vi "Event Demo.vi"() -> ()   [LabVIEW 2020]
uses:
  Flex/Flex.lvlib
  Flex/Element.ctl
  Flex/Event Data.ctl
panel:
  in  "Stop":bool
  in  "Slide":dbl(slide) scale=0.0..10.0
  out "Chart":dbl(graph)
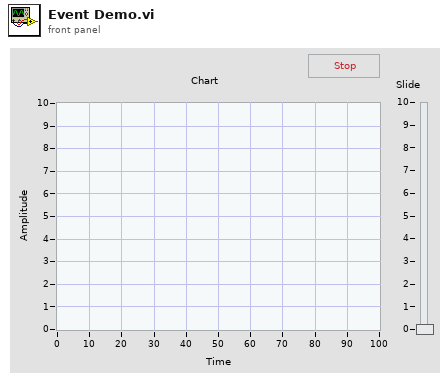
[diagram p1: front panel]
types:
  T1 = typedef "Flex.lvlib/))Channel.ctl" = refnum<queue>
  T2 = typedef "Flex.lvlib/Element.ctl" = dbl
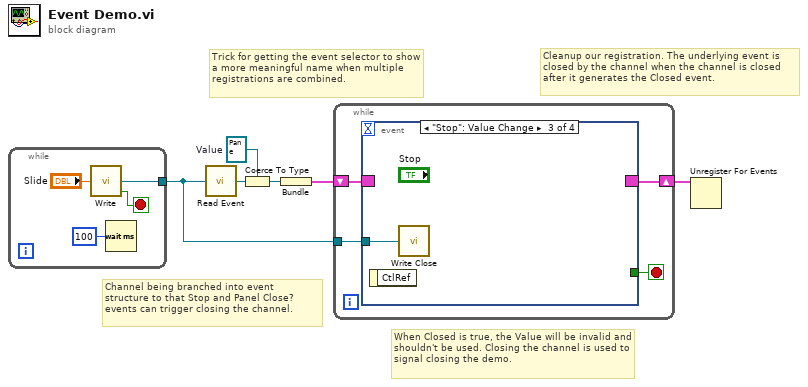
[diagram p0: block diagram]
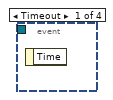
[diagram p2: hidden frame]
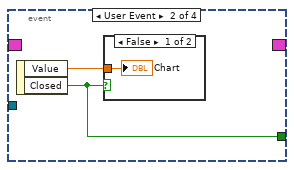
[diagram p3: hidden frame]
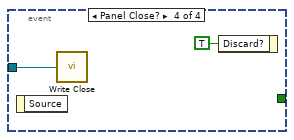
[diagram p5: hidden frame]
diagram:
  w4 = refnum<event-registration> refnum  # Value
  # "Cleanup our registration. The underlying event is closed by the channel when the channel is closed after it generates the Closed event."
  # "When Closed is true, the Value will be invalid and shouldn't be used. Closing the channel is used to signal closing the demo."
  # "Channel being branched into event structure to that Stop and Panel Close? events can trigger closing the channel."
  # "Trick for getting the event selector to show a more meaningful name when multiple registrations are combined."
  n1 = while {
    tunnel: [w10] -> w2
    stop <- w7 stop-if-true
    n2 = call "Write.vi"("element"="Slide") -> ("channel"=w10:T1, "Closed?"=w7:bool)  [unwired: 6 in, 1 out]
    n3 = Wait (ms)(milliseconds to wait=u32 100) -> ()  [unwired: 1 out]
  }
  n4 = call "Read Event.vi"("FlexChannel"=w2) -> ("Event Reg"=w6:refnum<event-registration>)  [unwired: 8 in]
  n5 = Coerce To Type(0:w6, 1:w4) -> (2:w5:refnum<event-registration>)
  n6 = Bundle("Value"=w5) -> (w3:cluster{"Value":refnum<event-registration>})  [unwired: 1 in]
  n7 = while {
    shift-right: [w13] -> w1
    shift-left: w3 -> [w14]
    tunnel: w2 -> [w11]
    stop <- w12 stop-if-true
    n8 = event shown="[2] \"Stop\": Value Change" {
      selector: w14 -> [_ _ _ _]
      dyn-events: [_ _ _ _] -> w13
      timeout: _ -> [_ _ _ _]
      tunnel: [_ w16 _ _] -> w12
      tunnel: w11 -> [_ _ w18 w19]
      event Timeout {
        n9 = event-data() -> ()  [unwired: 1 in, 1 out]
      }
      event User Event {
        n10 = event-data() -> ("Value"=w15:T2, "Closed"=w16:bool)  [unwired: 1 in]
        n11 = case shown="False" w16 {
          tunnel: w15 -> [w17 _]
          frame False {
            "Chart" <- w17
          }
          frame True {
          }
        }
      }
      event "Stop": Value Change {
        n12 = event-data() -> ()  [unwired: 1 in, 1 out]
        n13 = call "Write Close.vi"("FlexChannel"=w18) -> ()
      }
      event Panel Close? {
        n14 = event-data() -> ()  [unwired: 1 in, 1 out]
        n15 = call "Write Close.vi"("FlexChannel"=w19) -> ()
        n16 = event-data("Discard?"=TRUE) -> ()  [unwired: 1 in, 1 out]
      }
    }
  }
  n17 = Unregister For Events(event registration refnum=w1) -> ()  [unwired: 1 in, 1 out]
